vi "SafetyAccess.vi"(0 "Operation Interface in":refnum<class "Operation Interface.lvclass">, 1 "Robot Status":T1, 5 "error in (no error)":errorcluster) -> (14 "Operation Interface out":refnum<class "Operation Interface.lvclass">, 19 "error out":errorcluster)   [LabVIEW 2016, in "Operation Interface.lvclass"]
uses:
  Operation Interface.lvclass
  Universal Robot/RobotStatus.ctl
  Universal Robot/RobotMode.ctl
  Universal Robot/OperationalMode.ctl
  Universal Robot/SafetyStatus.ctl
  Operation Interface.lvclass/Operation Interface.ctl
  Universal Robot/Universal Robot.lvclass
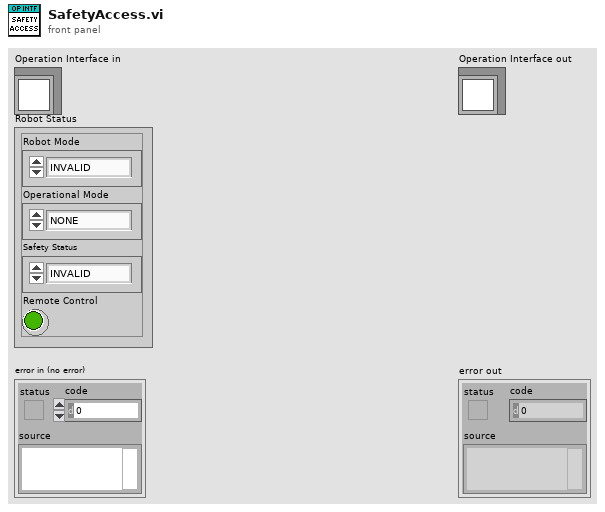
[diagram p1: front panel]
types:
  T1 = typedef "Universal Robot.lvclass/RobotStatus.ctl" = cluster{"Robot Mode":T2, "Operational Mode":T3, "Safety Status":T4, "Remote Control":bool}
  T2 = typedef "Universal Robot.lvclass/RobotMode.ctl" = enum16{"INVALID", "NO_CONTROLLER", "DISCONNECTED", "CONFIRM_SAFETY", "BOOTING", "POWER_OFF", "POWER_ON", "IDLE", "BACKDRIVE", "RUNNING"}
  T3 = typedef "Universal Robot.lvclass/OperationalMode.ctl" = enum16{"NONE", "MANUAL", "AUTOMATIC"}
  T4 = typedef "Universal Robot.lvclass/SafetyStatus.ctl" = enum16{"INVALID", "NORMAL", "REDUCED", "PROTECTIVE_STOP", "RECOVERY", "SAFEGAURD_STOP", "SYSTEM_EMERGENCY_STOP", "ROBOT_EMERGENCY_STOP", "VIOLATION", "FAULT", "AUTOMATIC_MODE_SAFEGAURD_STOP", "SYSTEM_THREE_POSITION_ENABLING_STOP"}
  T5 = enum8{"Enabled", "Disabled", "Disabled and Grayed Out"}
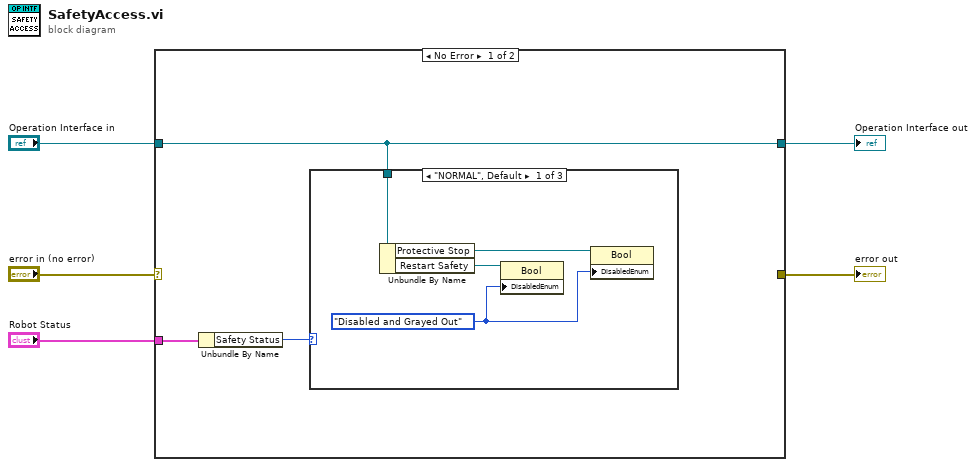
[diagram p0: block diagram]
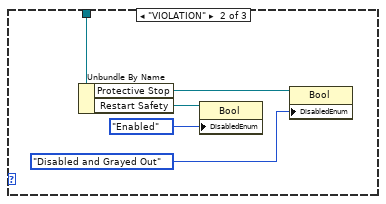
[diagram p2: hidden frame]
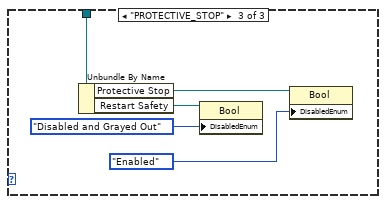
[diagram p3: hidden frame]
diagram:
  n1 = case shown="No Error" "error in (no error)" {
    selector: "error in (no error)" -> [_ w24]
    tunnel: [_ w24] -> w4
    tunnel: [w8 w23] -> w2
    tunnel: "Operation Interface in" -> [w8 w23]
    tunnel: "Robot Status" -> [w7 _]
    frame No Error {
      n2 = Unbundle By Name(w7) -> ("Safety Status"=w6:T4)
      n3 = case shown="\"NORMAL\", Default" w6 {
        tunnel: w8 -> [w12 w17 w22]
        frame "NORMAL", Default {
          w9 = T5."Disabled and Grayed Out" ("Disabled")
          n4 = Unbundle By Name(w12) -> ("Protective Stop"=w10:refnum<vi>, "Restart Safety"=w11:refnum<vi>)
          n5 = property class="Bool"(reference=w11, "DisabledEnum"=w9) -> ()  [unwired: 1 in, 2 out]
          n6 = property class="Bool"(reference=w10, "DisabledEnum"=w9) -> ()  [unwired: 1 in, 2 out]
        }
        frame "VIOLATION" {
          n7 = Unbundle By Name(w17) -> ("Protective Stop"=w15:refnum<vi>, "Restart Safety"=w16:refnum<vi>)
          n8 = property class="Bool"(reference=w16, "DisabledEnum"=T5."Enabled" ("Disabled")) -> ()  [unwired: 1 in, 2 out]
          n9 = property class="Bool"(reference=w15, "DisabledEnum"=T5."Disabled and Grayed Out" ("Disabled")) -> ()  [unwired: 1 in, 2 out]
        }
        frame "PROTECTIVE_STOP" {
          n10 = Unbundle By Name(w22) -> ("Protective Stop"=w20:refnum<vi>, "Restart Safety"=w21:refnum<vi>)
          n11 = property class="Bool"(reference=w21, "DisabledEnum"=T5."Disabled and Grayed Out" ("Disabled")) -> ()  [unwired: 1 in, 2 out]
          n12 = property class="Bool"(reference=w20, "DisabledEnum"=T5."Enabled" ("Disabled")) -> ()  [unwired: 1 in, 2 out]
        }
      }
    }
    frame Error {
    }
  }
  "error out" <- w4
  "Operation Interface out" <- w2
